vi "Rotation stage shgv5.vi"() -> ()   [LabVIEW 2020]
doc: "Shows how to move a motor to an absolute position."
uses:
  <vilib>/DAQmx/configure/timing.llb/DAQmx Timing (Implicit).vi
  <resource>/objmgr/daqmx.rc
  <vilib>/Utility/error.llb/DialogType.ctl
  <vilib>/DAQmx/read.llb/DAQmx Read (Counter 1D U32 1Chan NSamp).vi
  <vilib>/DAQmx/read.llb/DAQmx Read (Analog 1D Wfm NChan 1Samp).vi
  <vilib>/DAQmx/configure/timing.llb/DAQmx Timing (Sample Clock).vi
  <vilib>/DAQmx/create/channels.llb/DAQmx Create Channel (AI-Current-Basic).vi
  <vilib>/DAQmx/create/channels.llb/DAQmx Create Channel (CI-Period).vi
  <vilib>/DAQmx/create/channels.llb/DAQmx Create Channel (CO-Pulse Generation-Frequency).vi
panel:
  out "Actual Sample Rate":dbl=1000.0 format="%0.2f"
  out "data 2":waveform(dbl)[](graph)
  out "Consumer Iteration 3":i32=1109257
  in  "stop 4":bool
  out "Producer Iteration 3":i32=1109256
  out "error out 3":errorcluster
  out "Loop Time (ms) 3":u32=10
  in  "Duty Cycle":dbl=0.5 format="%.6f"
  out "Input.BufSize":u32=1000000 format="%.0p"
  out "data":u32[](graph)
  out "Consumer Iteration 2":i32=1109257
  in  "stop 3":bool
  in  "number of samples per channel 2":i32=5000
  out "Producer Iteration 2":i32=1109256
  out "error out 2":errorcluster
  out "Loop Time (ms) 2":u32=10
  in  "dwell time (ms)":dbl=1.0 format="%.6f"
  in  "Photon Input (PFI)":tag="/Dev1/PFI0"
  in  "Rotation Angle (Degrees)":dbl=100.0 min=0.0
  in  "MG17Motor":refnum<k7>(container)
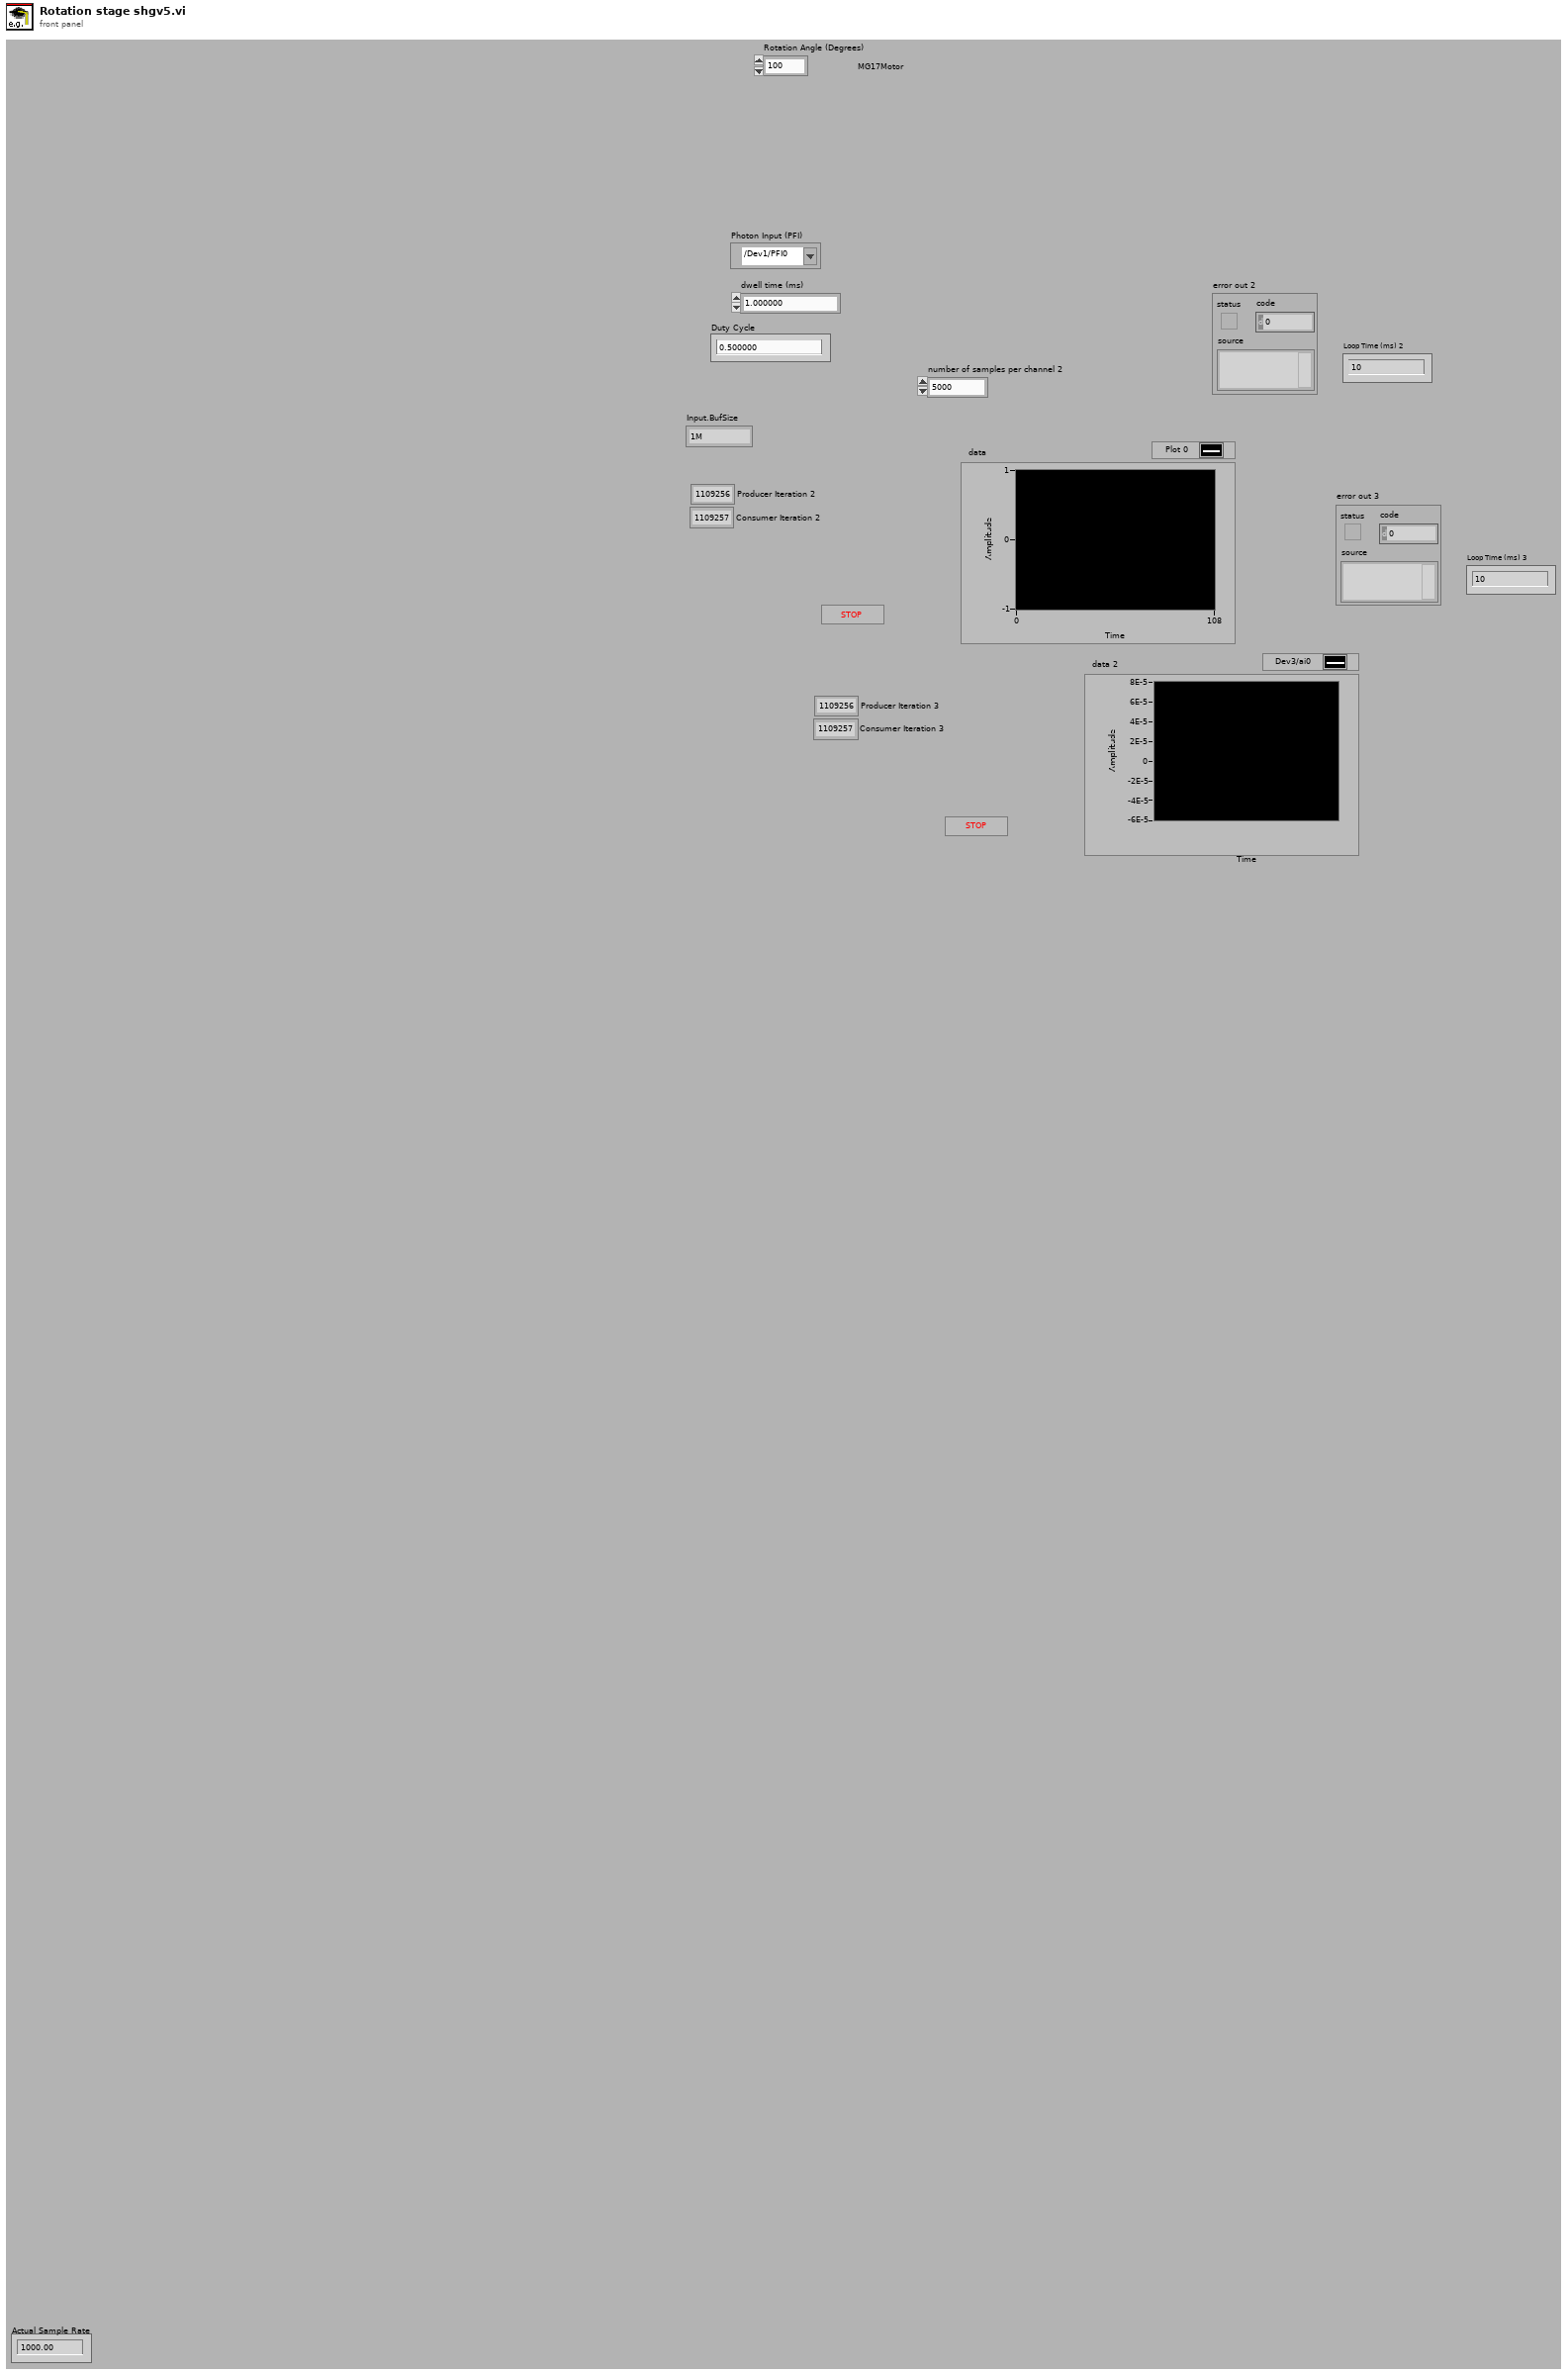
[diagram p1: front panel]
types:
  T1 = enum16{"open", "open or create", "create or replace", "create", "open (read-only)"}
  T2 = typedef "DialogType.ctl" = u16
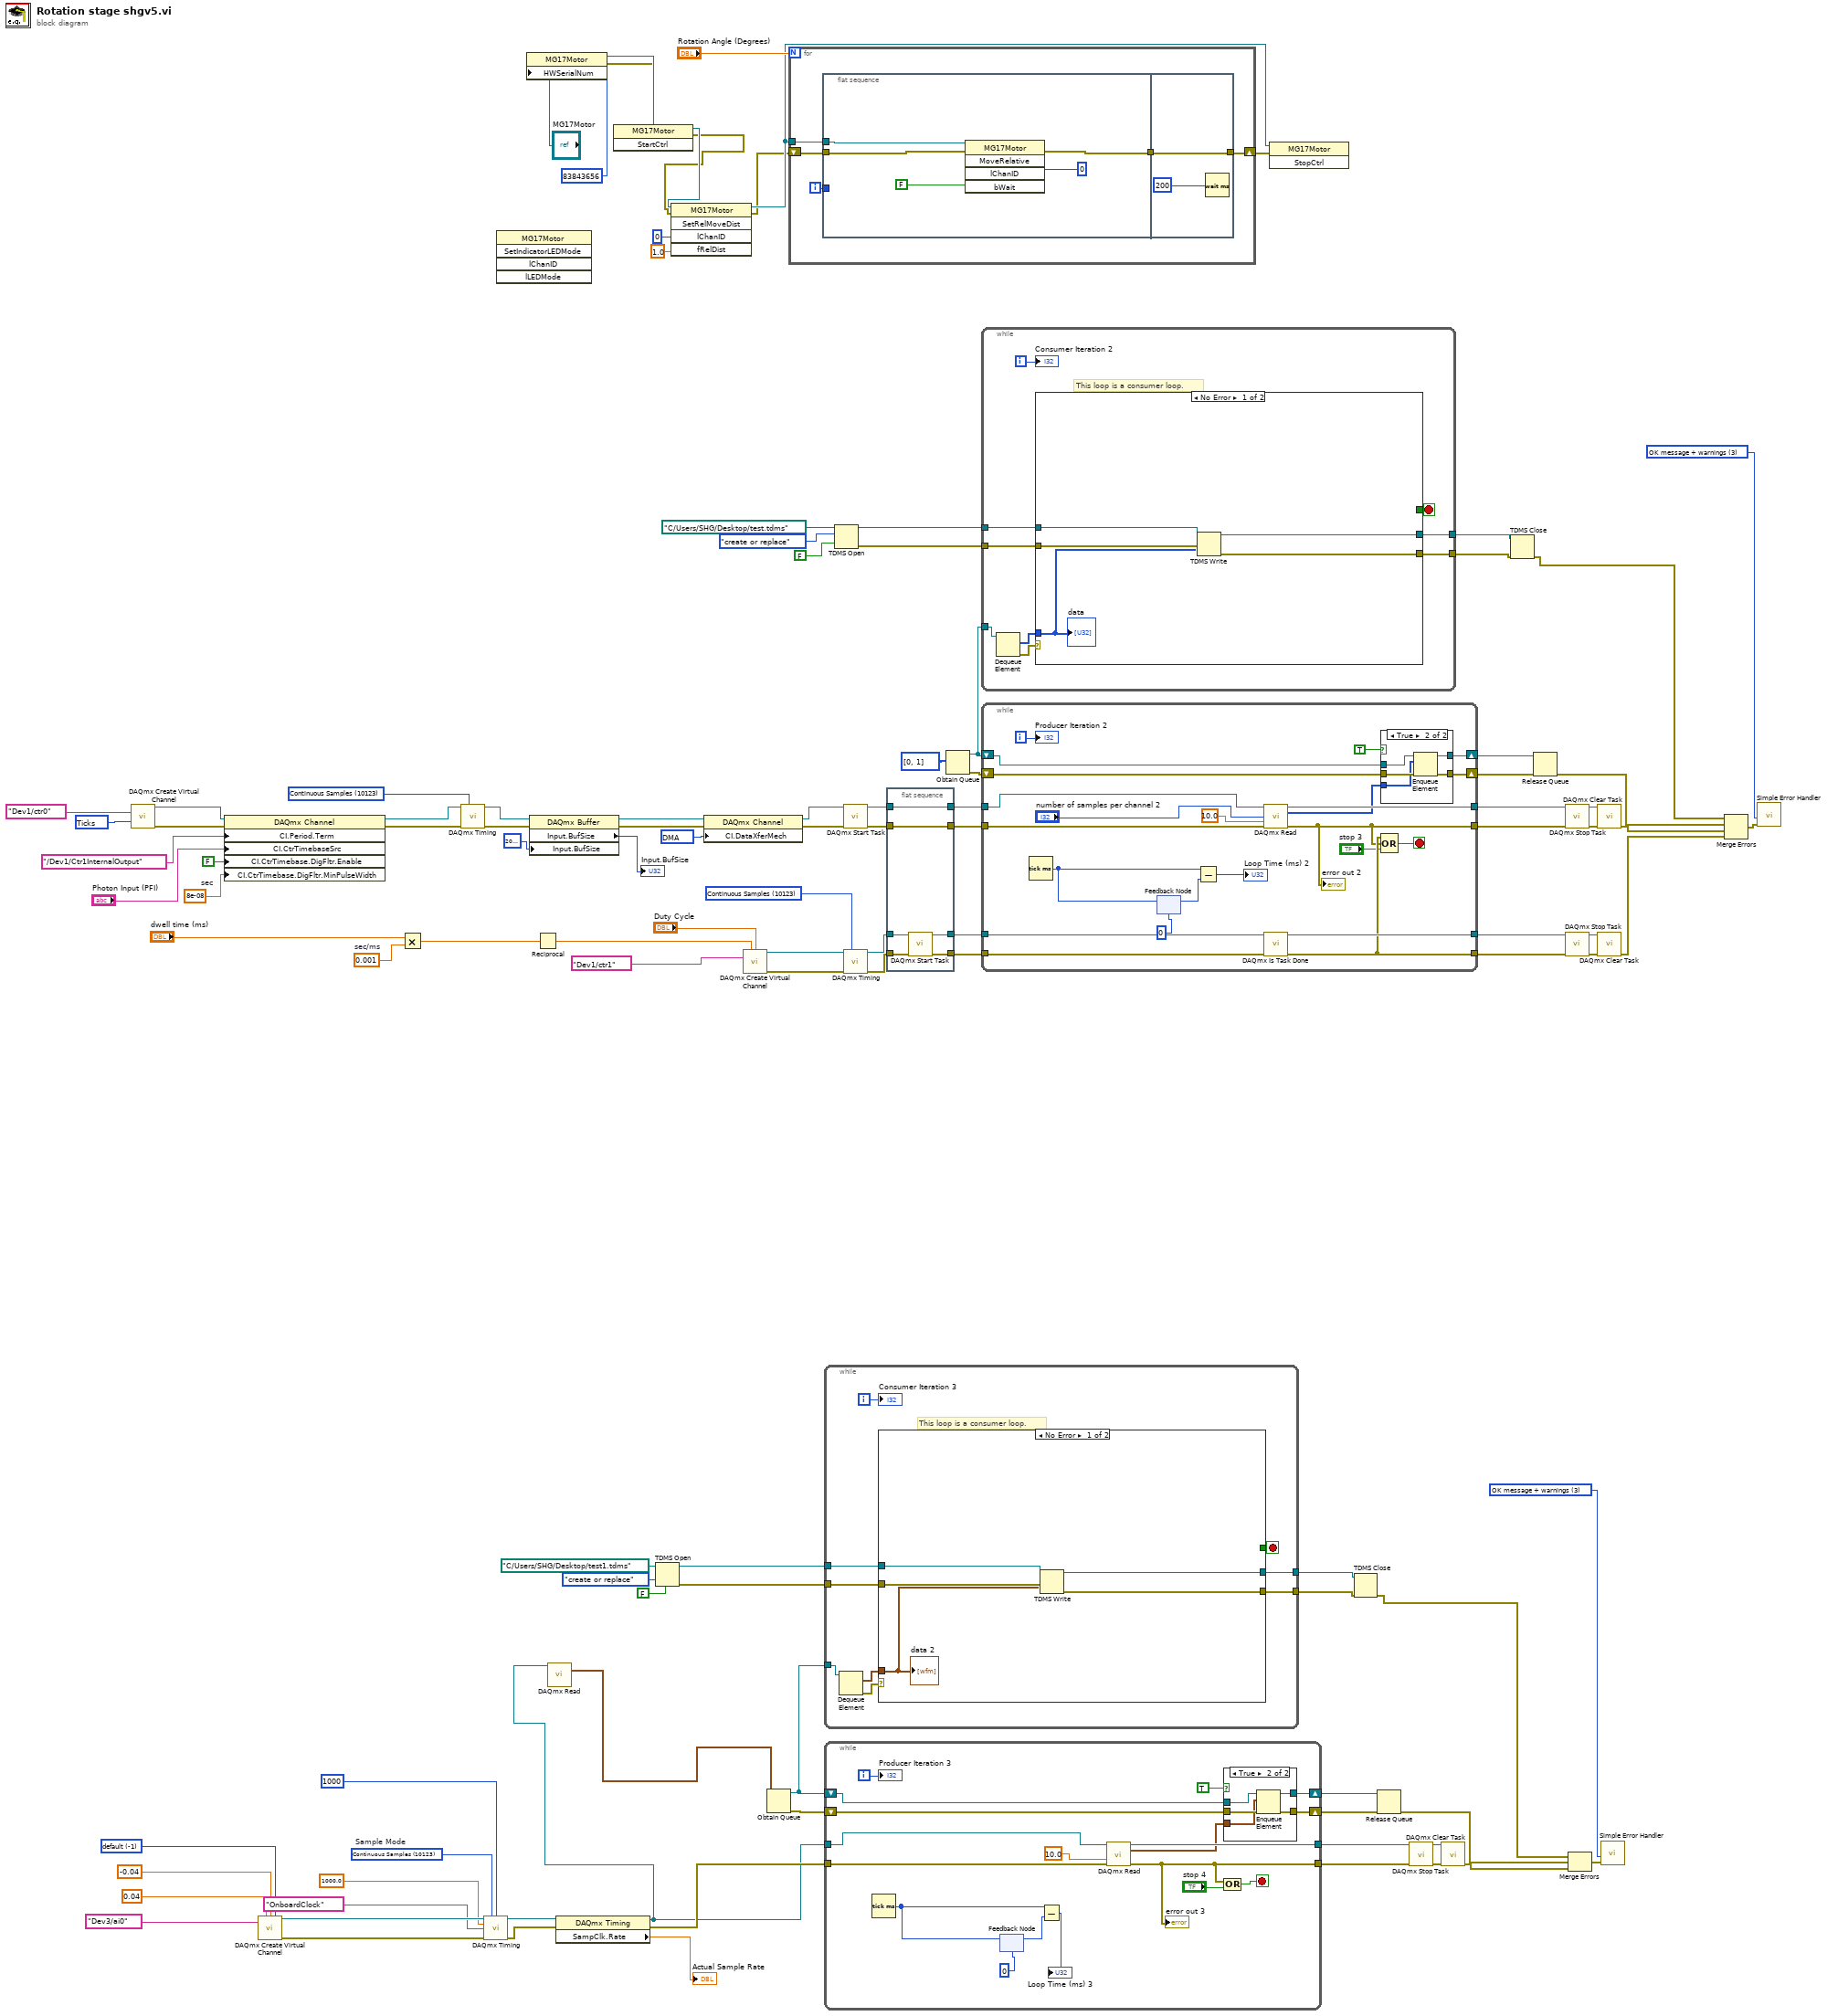
[diagram p0: block diagram]
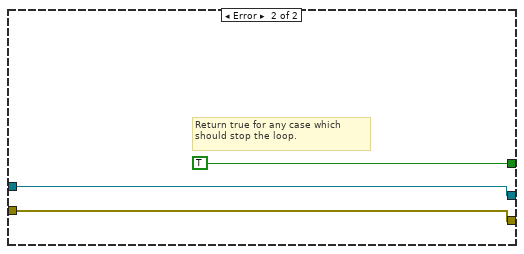
[diagram p2: hidden frame]
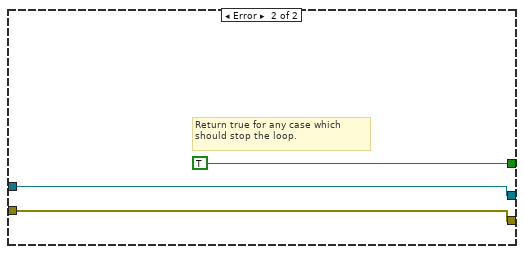
[diagram p4: hidden frame]
diagram:
  w12 = -1 items=["default"=-1, "RSE"=10083, "NRSE"=10078, "Differential"=10106, "Pseudodifferential"=12529] ("Terminal Configuration")
  w20 = 10123 items=["Finite Samples"=10178, "Continuous Samples"=10123, "Hardware Timed Single Point"=12522]  # Sample Mode
  w30 = T2 3 items=["no dialog", "OK message", "continue or stop message", "OK message + warnings", "continue/stop + warnings"] ("type of dialog (OK msg:1)")
  w51 = T2 3 items=["no dialog", "OK message", "continue or stop message", "OK message + warnings", "continue/stop + warnings"] ("type of dialog (OK msg:1)")
  w56 = 8e-08  # sec
  w67 = 10054 items=["DMA"=10054, "Interrupts"=10204, "Programmed I/O"=10264, "USB Bulk"=12590] ("CI.DataXferMech")
  w87 = 0.001  # sec/ms
  w97 = 10304 items=["Seconds"=10364, "Ticks"=10304, "From Custom Scale"=10065] ("units")
  w98 = 10123 items=["Finite Samples"=10178, "Continuous Samples"=10123, "Hardware Timed Single Point"=12522] ("sample mode")
  w99 = 10123 items=["Finite Samples"=10178, "Continuous Samples"=10123, "Hardware Timed Single Point"=12522] ("sample mode")
  n1 = call-poly <vilib>:"DAQmx Create Virtual Channel.vi"("counter"=tag "Dev1/ctr0", "units"=w97) -> ("task out"=w94:refnum<k21>, "error out"=w93:errorcluster)  [unwired: 12 in]
  n2 = property class="DAQmx Channel"(reference=w94, error in=w93, "CI.Period.Term"=tag "/Dev1/Ctr1InternalOutput", "CI.CtrTimebaseSrc"="Photon Input (PFI)", "CI.CtrTimebase.DigFltr.Enable"=FALSE, "CI.CtrTimebase.DigFltr.MinPulseWidth"=w56) -> (reference out=w92:refnum<k21>, error out=w91:errorcluster)
  n3 = call-poly <vilib>:"DAQmx Create Virtual Channel.vi"("maximum value"=0.04 ("Max Voltage"), "minimum value"=-0.04 ("Min Voltage"), "input terminal configuration"=w12, "physical channels"=tag "Dev3/ai0" ("Physical Channel")) -> ("task out"=w18:refnum<k21>, "error out"=w19:errorcluster)  [unwired: 10 in]
  n4 = Multiply(x="dwell time (ms)", y=w87) -> (x*y=w86:dbl)
  n5 = call-poly <vilib>:"DAQmx Timing.vi"("task/channels in"=w92, "sample mode"=w98, "error in"=w91) -> ("task out"=w62:refnum<k21>, "error out"=w61:errorcluster)  [unwired: 11 in]
  n6 = call-poly <vilib>:"DAQmx Timing.vi"("task/channels in"=w18, "sample mode"=w20, "samples per channel"=1000 ("Number of Samples"), "rate"=1000.0 ("Sample Rate"), "source"=tag "OnboardClock" ("Sample Clock Source"), "error in"=w19) -> ("task out"=w22:refnum<k21>, "error out"=w21:errorcluster)  [unwired: 8 in]
  n7 = invoke class="MG17Motor" method="SetIndicatorLEDMode"() -> ()  [unwired: 5 in, 5 out]
  n8 = property class="MG17Motor"(reference="MG17Motor", "HWSerialNum"=83843656) -> (reference out=w109:refnum<k7>, error out=w108:errorcluster)  [unwired: 1 in]
  n9 = property class="DAQmx Buffer"(reference=w62, error in=w61, "Input.BufSize"=u32 2000000 ("samples per channel")) -> (reference out=w66:refnum<k21>, error out=w64:errorcluster, "Input.BufSize"=→"Input.BufSize":u32)
  n10 = Reciprocal(x=w86) -> (1/x=w85:dbl)
  n11 = property class="DAQmx Timing"(reference=w22, error in=w21) -> (reference out=w7:refnum<k21>, error out=w16:errorcluster, "SampClk.Rate"=→"Actual Sample Rate":dbl)
  n12 = call-poly <vilib>:"DAQmx Read.vi"("task/channels in"=w7) -> ("data"=w8:waveform(dbl)[])  [unwired: 12 in, 2 out]
  n13 = invoke class="MG17Motor" method="StartCtrl"(reference=w109, error in=w108) -> (reference out=w4:refnum<k7>, error out=w2:errorcluster)  [unwired: 1 in, 1 out]
  n14 = TDMS Open(6:FALSE ("disable buffering? (T)"), 10:T1."create or replace" ("operation (0:open)"), 11:path "C:/Users/SHG/Desktop/test1.tdms" ("file path")) -> (0:w32:errorcluster, 3:w34:refnum<k34>)  [unwired: 4 in]
  n15 = invoke class="MG17Motor" method="SetRelMoveDist"(reference=w4, error in=w2, "lChanID"=0, "fRelDist"=sgl 1.0) -> (reference out=w3:refnum<k7>, error out=w1:errorcluster)  [unwired: 1 in, 3 out]
  n16 = property class="DAQmx Channel"(reference=w66, error in=w64, "CI.DataXferMech"=w67) -> (reference out=w60:refnum<k21>, error out=w59:errorcluster)
  n17 = call-poly <vilib>:"DAQmx Create Virtual Channel.vi"("frequency"=w85, "duty cycle"="Duty Cycle", "counter"=tag "Dev1/ctr1") -> ("task out"=w104:refnum<k21>, "error out"=w105:errorcluster)  [unwired: 11 in]
  n18 = Obtain Queue(element data type=w8) -> (queue out=w42:refnum<queue>, error out=w41:errorcluster)  [unwired: 4 in, 1 out]
  n19 = for {
    N: "Rotation Angle (Degrees)" -> [_]
    tunnel: w3 -> [w116]
    shift-right: [w114] -> w111
    shift-left: w1 -> [w115]
    i -> [w112]
    n20 = flat-sequence {
      tunnel: w116 -> [w121]
      tunnel: w115 -> [w120]
      tunnel: [w119] -> w113
      tunnel: w112 -> [_]
      tunnel: [w123] -> w114
      tunnel: w113 -> [w123]
      frame #0 {
        n21 = invoke class="MG17Motor" method="MoveRelative"(reference=w121, error in=w120, "lChanID"=0, "bWait"=FALSE) -> (error out=w119:errorcluster)  [unwired: 1 in, 4 out]
      }
      frame #1 {
        n22 = Wait (ms)(milliseconds to wait=u32 200) -> ()  [unwired: 1 out]
      }
    }
  }
  n23 = while {
    tunnel: w42 -> [w132]
    tunnel: w34 -> [w127]
    tunnel: [w126] -> w33
    tunnel: w32 -> [w125]
    tunnel: [w124] -> w31
    i -> [w128]
    stop <- w129 stop-if-true
    # "This loop is a consumer loop."
    n24 = Dequeue Element(queue=w132) -> (element=w130:waveform(dbl)[], error out=w131:errorcluster)  [unwired: 2 in, 2 out]
    n25 = case shown="No Error" w131 {
      tunnel: w130 -> [w133 _]
      tunnel: [_ TRUE] -> w129
      tunnel: w127 -> [w137 w139]
      tunnel: [w136 w139] -> w126
      tunnel: w125 -> [w135 w138]
      tunnel: [w134 w138] -> w124
      frame No Error {
        n26 = TDMS Write(0:w137, 9:w133, 11:w135) -> (4:w136:refnum<k34>, 15:w134:errorcluster)  [unwired: 3 in, 2 out]
        "data 2" <- w133
      }
      frame Error {
        # "Return true for any case which should stop the loop."
      }
    }
    "Consumer Iteration 3" <- w128
  }
  n27 = while {
    shift-right: [w148] -> w39
    shift-left: w41 -> [w156]
    shift-right: [w157] -> w40
    shift-left: w42 -> [w158]
    tunnel: [w154] -> w36
    tunnel: [w147] -> w35
    tunnel: w16 -> [w153]
    tunnel: w7 -> [w152]
    i -> [w149]
    stop <- w145 stop-if-true
    n28 = Tick Count (ms)() -> (millisecond timer value=w144:u32)
    n29 = feedback #1(u32 0 ("millisecond timer value")) -> (w143:u32)
    n30 = feedback-in #1(w144) -> ()
    n31 = Subtract(x=w144, y=w143) -> (x-y=→"Loop Time (ms) 3":u32)
    n32 = call-poly <vilib>:"DAQmx Read.vi"("task/channels in"=w152, "timeout"=10.0, "error in"=w153) -> ("task out"=w154:refnum<k21>, "data"=w151:waveform(dbl)[], "error out"=w147:errorcluster)  [unwired: 10 in]
    "error out 3" <- w147
    n33 = case shown="True" TRUE ("Case Constant\n(See Context Help)") {
      tunnel: w158 -> [w160 w165]
      tunnel: [w160 w164] -> w157
      tunnel: w156 -> [w159 w163]
      tunnel: [w159 w162] -> w148
      tunnel: w151 -> [_ w161]
      frame False {
      }
      frame True {
        n34 = Enqueue Element(queue=w165, element=w161, error in (no error)=w163) -> (queue out=w164:refnum<queue>, error out=w162:errorcluster)  [unwired: 1 in, 1 out]
      }
    }
    n35 = Compound Arithmetic op=OR(w147, "stop 4") -> (w145:bool)
    "Producer Iteration 3" <- w149
  }
  n36 = TDMS Open(6:FALSE ("disable buffering? (T)"), 10:T1."create or replace" ("operation (0:open)"), 11:path "C:/Users/SHG/Desktop/test.tdms" ("file path")) -> (0:w53:errorcluster, 3:w55:refnum<k34>)  [unwired: 4 in]
  n37 = call <vilib>:"DAQmx Start Task.vi"("task/channels in"=w60, "error in"=w59) -> ("task out"=w84:refnum<k21>, "error out"=w83:errorcluster)  [unwired: 12 in]
  n38 = call-poly <vilib>:"DAQmx Timing.vi"("task/channels in"=w104, "sample mode"=w99, "error in"=w105) -> ("task out"=w103:refnum<k21>, "error out"=w102:errorcluster)  [unwired: 11 in]
  n39 = flat-sequence {
    tunnel: w103 -> [w171]
    tunnel: w102 -> [w170]
    tunnel: [w169] -> w70
    tunnel: [w168] -> w71
    tunnel: w84 -> [w166]
    tunnel: w83 -> [w167]
    tunnel: [w167] -> w73
    tunnel: [w166] -> w72
    frame #0 {
      n40 = call <vilib>:"DAQmx Start Task.vi"("task/channels in"=w171, "error in"=w170) -> ("task out"=w168:refnum<k21>, "error out"=w169:errorcluster)  [unwired: 12 in]
    }
  }
  n41 = Obtain Queue(element data type=u32[] [0, 1] ("data")) -> (queue out=w82:refnum<queue>, error out=w81:errorcluster)  [unwired: 4 in, 1 out]
  n42 = while {
    tunnel: w82 -> [w180]
    tunnel: w55 -> [w175]
    tunnel: [w174] -> w54
    tunnel: w53 -> [w173]
    tunnel: [w172] -> w52
    i -> [w176]
    stop <- w177 stop-if-true
    # "This loop is a consumer loop."
    n43 = Dequeue Element(queue=w180) -> (element=w178:u32[], error out=w179:errorcluster)  [unwired: 2 in, 2 out]
    n44 = case shown="No Error" w179 {
      tunnel: w178 -> [w181 _]
      tunnel: [_ TRUE] -> w177
      tunnel: w175 -> [w185 w187]
      tunnel: [w184 w187] -> w174
      tunnel: w173 -> [w183 w186]
      tunnel: [w182 w186] -> w172
      frame No Error {
        n45 = TDMS Write(0:w185, 9:w181, 11:w183) -> (4:w184:refnum<k34>, 15:w182:errorcluster)  [unwired: 3 in, 2 out]
        "data" <- w181
      }
      frame Error {
        # "Return true for any case which should stop the loop."
      }
    }
    "Consumer Iteration 2" <- w176
  }
  n46 = while {
    shift-right: [w200] -> w79
    shift-left: w81 -> [w209]
    shift-right: [w210] -> w80
    shift-left: w82 -> [w211]
    tunnel: [w207] -> w76
    tunnel: [w195] -> w75
    tunnel: w73 -> [w206]
    tunnel: w72 -> [w205]
    tunnel: w71 -> [w199]
    tunnel: w70 -> [w198]
    tunnel: [w197] -> w69
    tunnel: [w196] -> w68
    i -> [w201]
    stop <- w193 stop-if-true
    n47 = Tick Count (ms)() -> (millisecond timer value=w192:u32)
    n48 = feedback #2(u32 0 ("millisecond timer value")) -> (w191:u32)
    n49 = feedback-in #2(w192) -> ()
    n50 = Subtract(x=w192, y=w191) -> (x-y=→"Loop Time (ms) 2":u32)
    n51 = call-poly <vilib>:"DAQmx Read.vi"("task/channels in"=w205, "number of samples per channel"="number of samples per channel 2", "timeout"=10.0, "error in"=w206) -> ("task out"=w207:refnum<k21>, "data"=w204:u32[], "error out"=w195:errorcluster)  [unwired: 9 in]
    "error out 2" <- w195
    n52 = call <vilib>:"DAQmx Is Task Done.vi"("task/channels in"=w199, "error in"=w198) -> ("task out"=w197:refnum<k21>, "error out"=w196:errorcluster)  [unwired: 11 in, 1 out]
    n53 = case shown="True" TRUE ("Case Constant\n(See Context Help)") {
      tunnel: w211 -> [w213 w218]
      tunnel: [w213 w217] -> w210
      tunnel: w209 -> [w212 w216]
      tunnel: [w212 w215] -> w200
      tunnel: w204 -> [_ w214]
      frame False {
      }
      frame True {
        n54 = Enqueue Element(queue=w218, element=w214, error in (no error)=w216) -> (queue out=w217:refnum<queue>, error out=w215:errorcluster)  [unwired: 1 in, 1 out]
      }
    }
    n55 = Compound Arithmetic op=OR(w196, w195, "stop 3") -> (w193:bool)
    "Producer Iteration 2" <- w201
  }
  n56 = invoke class="MG17Motor" method="StopCtrl"(reference=w3, error in=w111) -> ()  [unwired: 1 in, 3 out]
  n57 = TDMS Close(8:w31, 11:w33) -> (0:w26:errorcluster)  [unwired: 1 out]
  n58 = Release Queue(queue=w40, error in (no error)=w39) -> (error out=w25:errorcluster)  [unwired: 1 in, 2 out]
  n59 = call <vilib>:"DAQmx Stop Task.vi"("task/channels in"=w36, "error in"=w35) -> ("task out"=w37:refnum<k21>, "error out"=w38:errorcluster)  [unwired: 12 in]
  n60 = call <vilib>:"DAQmx Clear Task.vi"("task in"=w37, "error in"=w38) -> ("error out"=w24:errorcluster)  [unwired: 13 in]
  n61 = TDMS Close(8:w52, 11:w54) -> (0:w47:errorcluster)  [unwired: 1 out]
  n62 = Release Queue(queue=w80, error in (no error)=w79) -> (error out=w46:errorcluster)  [unwired: 1 in, 2 out]
  n63 = call <vilib>:"DAQmx Stop Task.vi"("task/channels in"=w76, "error in"=w75) -> ("task out"=w77:refnum<k21>, "error out"=w78:errorcluster)  [unwired: 12 in]
  n64 = call <vilib>:"DAQmx Stop Task.vi"("task/channels in"=w69, "error in"=w68) -> ("task out"=w101:refnum<k21>, "error out"=w100:errorcluster)  [unwired: 12 in]
  n65 = Merge Errors(w26, w25, w24) -> (w29:errorcluster)
  n66 = call <vilib>:"DAQmx Clear Task.vi"("task in"=w77, "error in"=w78) -> ("error out"=w45:errorcluster)  [unwired: 13 in]
  n67 = call <vilib>:"DAQmx Clear Task.vi"("task in"=w101, "error in"=w100) -> ("error out"=w44:errorcluster)  [unwired: 13 in]
  n68 = call <vilib>:"Simple Error Handler.vi"("type of dialog (OK msg:1)"=w30, "error in (no error)"=w29) -> ()  [unwired: 3 in, 5 out]
  n69 = Merge Errors(w47, w46, w45, w44) -> (w50:errorcluster)
  n70 = call <vilib>:"Simple Error Handler.vi"("type of dialog (OK msg:1)"=w51, "error in (no error)"=w50) -> ()  [unwired: 3 in, 5 out]
